vi "init.vi"(8 "error in (no error)":errorcluster, 10 "Commands to run":string[](array[string]), 11 "VISA Refnum in":refnum<visa-resource-name>) -> (0 "error out":errorcluster, 3 "VISA Refnum out":refnum<visa-resource-name>)   [LabVIEW 2020]
uses:
  haltnow.vi
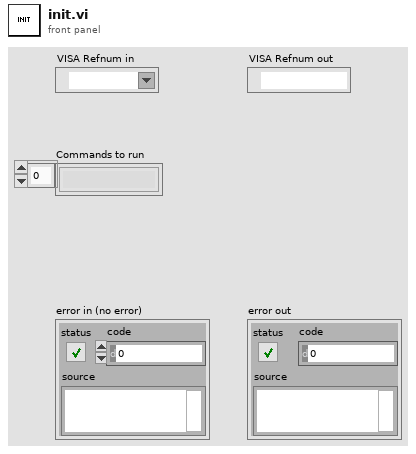
[diagram p1: front panel]
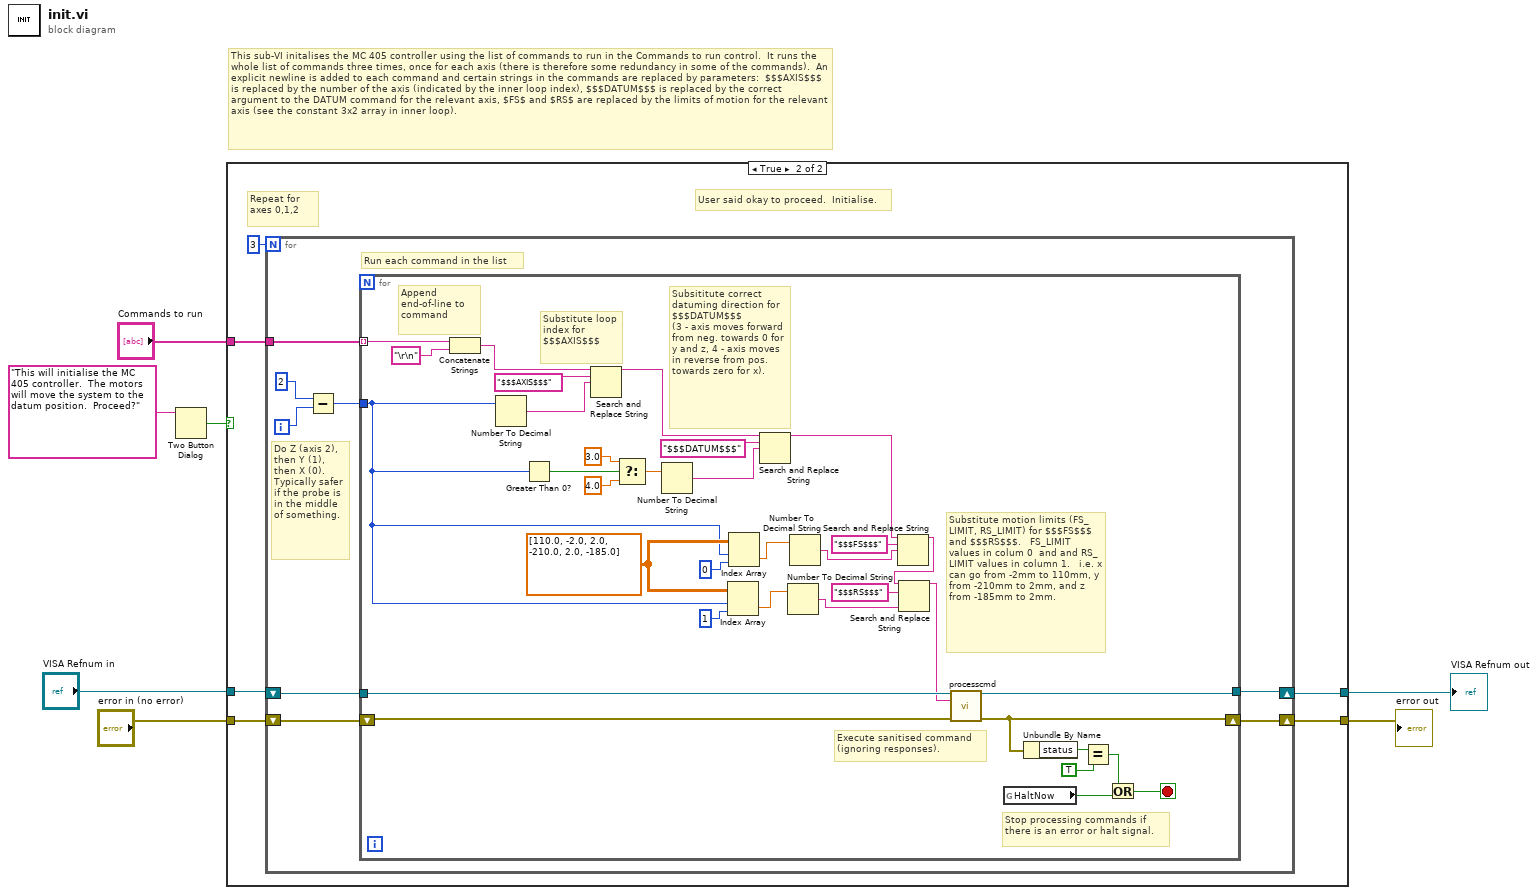
[diagram p0: block diagram]
diagram:
  # "This sub-VI initalises the MC 405 controller using the list of commands to run in the Commands to run control.  It runs the whole list of commands three times, once for each axis (there is therefore some redundancy in some of the commands).  An explicit newline is added to each command and certain strings in the commands are replaced by parameters:  $$$AXIS$$$ is replaced by the number of the axis (indicated by the inner loop index), $$$DATUM$$$ is replaced by the correct argument to the DATUM command for the relevant axis, $FS$ and $RS$ are replaced by the limits of motion for the relevant axis (see the constant 3x2 array in inner loop)."
  n1 = Two Button Dialog(message="This will initialise the MC 405 controller.  The motors will move the system to the datum position.  Proceed?") -> (T button?=w1:bool)  [unwired: 2 in]
  n2 = case shown="True" w1 {
    tunnel: [w9 w15] -> w6
    tunnel: "VISA Refnum in" -> [w9 w14]
    tunnel: "Commands to run" -> [_ w13]
    tunnel: [w8 w12] -> w3
    tunnel: "error in (no error)" -> [w8 w11]
    frame False {
      # "User said not okay to proceed.  Do nothing."
    }
    frame True {
      # "User said okay to proceed.  Initialise."
      # "Repeat for axes 0,1,2"
      n3 = for {
        N: 3 -> [_]
        tunnel: w13 -> [w21]
        shift-right: [w23] -> w15
        shift-left: w14 -> [w22]
        shift-right: [w20] -> w12
        shift-left: w11 -> [w19]
        i -> [w17]
        # "Do Z (axis 2), then Y (1), then X (0).  Typically safer if the probe is in the middle of something."
        # "Run each command in the list"
        n4 = Subtract(x=2, y=w17) -> (x-y=w16:i32)
        n5 = for {
          shift-right: [w52] -> w20
          shift-left: w19 -> [w57]
          tunnel: w21 -> [w53] mode=indexing
          tunnel: w22 -> [w56]
          tunnel: [w55] -> w23
          tunnel: w16 -> [w33]
          stop <- w44 stop-if-true
          w34 = dbl[][] [[110.0, -2.0], [2.0, -210.0], [2.0, -185.0]]
          # "Stop processing commands if there is an error or halt signal."
          # "Execute sanitised command\n(ignoring responses)."
          # "Subsititute correct datuming direction for $$$DATUM$$$ \n(3 - axis moves forward from neg. towards 0 for y and z, 4 - axis moves in reverse from pos. towards zero for x)."
          # "Substitute loop index for $$$AXIS$$$"
          # "Append end-of-line to command"
          # "Substitute motion limits (FS_LIMIT, RS_LIMIT) for $$$FS$$$ and $$$RS$$$.   FS_LIMIT values in colum 0  and and RS_LIMIT values in column 1.   i.e. x can go from -2mm to 110mm, y from -210mm to 2mm, and z from -185mm to 2mm."
          n6 = Concatenate Strings(w53, "\r\n" ("string")) -> (w48:string)
          n7 = Number To Decimal String(number=w33) -> (decimal integer string=w49:string)  [unwired: 1 in]
          n8 = Greater Than 0?(x=w33) -> (x > 0?=w43:bool)
          n9 = Search and Replace String(input string=w48, search string="$$$AXIS$$$", replace string=w49) -> (result string=w37:string)  [unwired: 5 in, 3 out]
          n10 = Select(t=3.0, s=w43, f=4.0) -> (s? t:f=w39:dbl)
          n11 = Number To Decimal String(number=w39) -> (decimal integer string=w38:string)  [unwired: 1 in]
          n12 = Index Array(array=w34, index (row)=w33, index (col)=1 ("disabled index (col)")) -> (element=w31:dbl)
          n13 = Index Array(array=w34, index (row)=w33, index (col)=0 ("disabled index (col)")) -> (element=w32:dbl)
          n14 = Search and Replace String(input string=w37, search string="$$$DATUM$$$", replace string=w38) -> (result string=w29:string)  [unwired: 5 in, 3 out]
          n15 = Number To Decimal String(number=w31) -> (decimal integer string=w25:string)  [unwired: 1 in]
          n16 = Number To Decimal String(number=w32) -> (decimal integer string=w26:string)  [unwired: 1 in]
          n17 = Search and Replace String(input string=w29, search string="$$$FS$$$", replace string=w26) -> (result string=w28:string)  [unwired: 5 in, 3 out]
          n18 = Search and Replace String(input string=w28, search string="$$$RS$$$" ("replace string (\"\")"), replace string=w25) -> (result string=w27:string)  [unwired: 5 in, 3 out]
          n19 = call "processcmd.vi"("VISA Refnum in"=w56, "write buffer"=w27, "error in (no error)"=w57) -> ("VISA Refnum out"=w55:refnum<visa-resource-name>, "error out"=w52:errorcluster)  [unwired: 10 in, 1 out]
          n20 = global read "haltnow.vi" "HaltNow"() -> (w46:bool)
          n21 = Unbundle By Name(w52) -> ("status"=w51:bool)
          n22 = Equal?(x=w51, y=TRUE) -> (x = y?=w45:bool)
          n23 = Or(x=w45, y=w46) -> (x .or. y?=w44:bool)
        }
      }
    }
  }
  "VISA Refnum out" <- w6
  "error out" <- w3
